vi "Authorization Write License File.vi"(8 "error in (no error)":errorcluster, 9 "Authorization":T1, 10 "Hardware ID":string, 11 "Spartan License File Path":path) -> (0 "error out":errorcluster)   [LabVIEW 2011]
uses:
  Authorization Data.ctl
panel:
  in  "Debug? (f)":bool
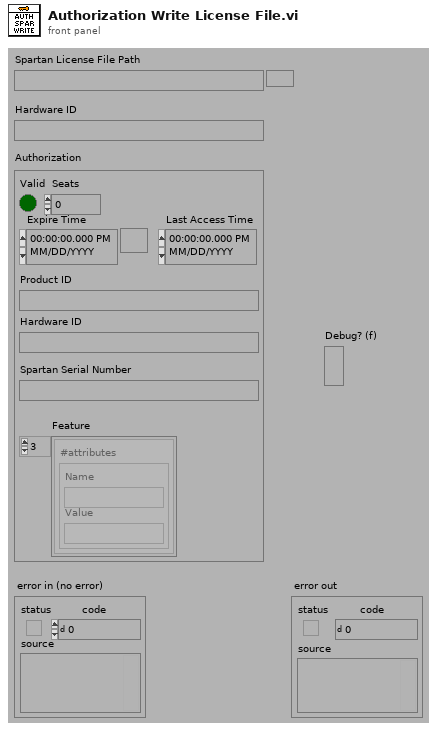
[diagram p1: front panel]
types:
  T1 = typedef "Authorization Data.ctl" = cluster{"Valid":bool, "Seats":i32, "Expire Time":timestamp, "Last Access Time":timestamp, "Product ID":string, "Hardware ID":string, "Spartan Serial Number":string, "Feature":cluster{"#attributes":cluster{"Name":string, "Value":string}}[]}
  T2 = cluster{"#attributes":cluster{"Name":string, "Value":string}}[]
  T3 = cluster{"#attributes":cluster{"Name":string, "Value":string}}
  T4 = enum16{"open", "replace", "create", "open or create", "replace or create", "replace or create with confirmation"}
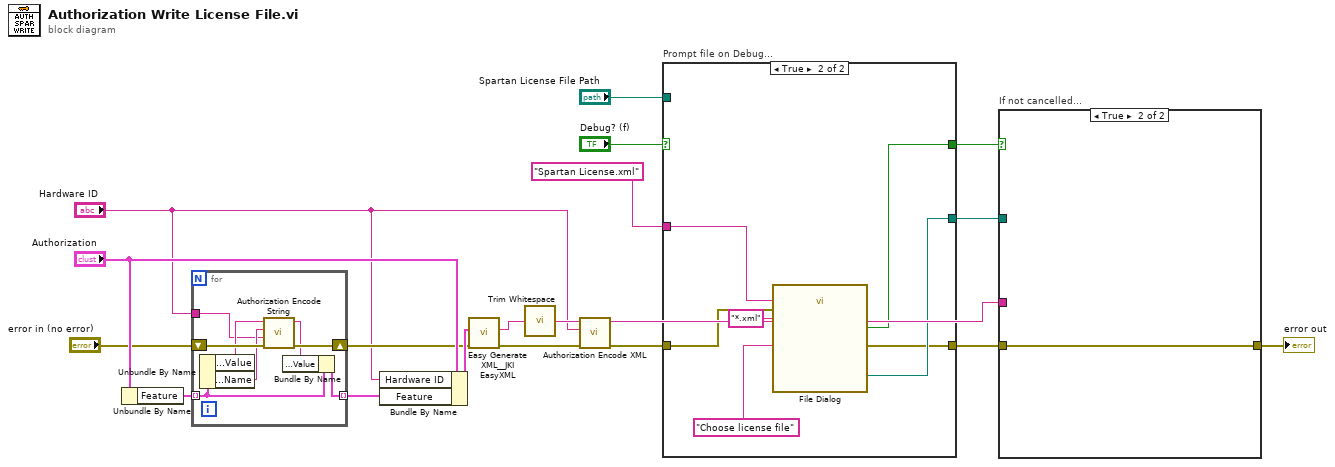
[diagram p0: block diagram]
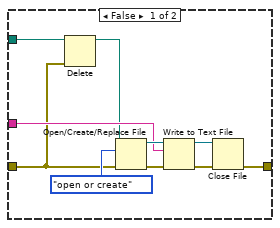
[diagram p2: hidden frame]
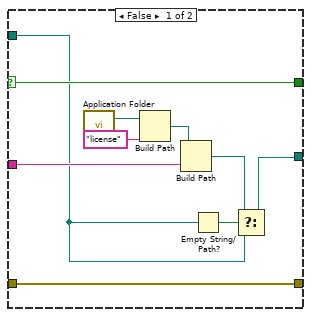
[diagram p3: hidden frame]
diagram:
  n1 = Unbundle By Name("Authorization") -> ("Feature"=w11:T2)
  n2 = for {
    tunnel: w11 -> [w26] mode=indexing
    tunnel: [w25] -> w10 mode=indexing
    shift-right: [w23] -> _
    shift-left: "error in (no error)" -> [w24]
    tunnel: "Hardware ID" -> [w19]
    n3 = Unbundle By Name(w26) -> ("#attributes.Value"=w21:string, "#attributes.Name"=w22:string)
    n4 = call "Authorization Encode String.vi"("error in (no error)"=w24, "Volume Serial Number"=w19, "Property Name"=w22, "Decoded String"=w21) -> ("error out"=w23:errorcluster, "Encoded String"=w20:string)  [unwired: 6 in]
    n5 = Bundle By Name(cluster=w26, "#attributes.Value"=w20) -> (w25:T3)
  }
  n6 = Bundle By Name(cluster="Authorization", "Hardware ID"="Hardware ID", "Feature"=w10) -> (w15:T1)
  n7 = call "Easy Generate XML__JKI EasyXML.vi"("error in (no error)"="error in (no error)", "LabVIEW Data"=w15) -> ("error out"=w18:errorcluster, "XML String"=w14:string)  [unwired: 8 in]
  n8 = call <vilib>:"Trim Whitespace.vi"("string"=w14) -> ("trimmed string"=w13:string)  [unwired: 1 in]
  n9 = call "Authorization Encode XML.vi"("error in (no error)"=w18, "Volume Serial Number"="Hardware ID", "Decoded XML String"=w13) -> ("error out"=w4:errorcluster, "Encoded XML String"=w16:string)  [unwired: 7 in]
  n10 = case "Prompt file on Debug..." shown="True" "Debug? (f)" {
    selector: "Debug? (f)" -> [w35 _]
    tunnel: [w28 w43] -> w2
    tunnel: "Spartan License.xml" ("Relative Path (\"\" - Folder)") -> [w31 w40]
    tunnel: [w36 w38] -> w3
    tunnel: w4 -> [w36 w39]
    tunnel: [w35 w37] -> w5
    tunnel: "Spartan License File Path" -> [w27 _]
    frame False {
      n11 = call "Application Folder.vi"() -> ("Application Folder"=w34:path)  [unwired: 3 in]
      n12 = Build Path(base path=w34, name or relative path="license" ("Relative Path (\"\" - Folder)")) -> (appended path=w32:path)
      n13 = Build Path(base path=w32, name or relative path=w31) -> (appended path=w29:path)
      n14 = Empty String/Path?(string/path=w27) -> (empty?=w30:bool)
      n15 = Select(t=w29, s=w30, f=w27) -> (s? t:f=w28:path)
    }
    frame True {
      n16 = call "File Dialog"("prompt"="Choose license file", "default name"=w40, "error in"=w39, "pattern (all files)"="*.xml") -> ("selected path"=w43:path, "cancelled"=w37:bool, "error out"=w38:errorcluster)  [unwired: 8 in, 1 out]
    }
  }
  n17 = case "If not cancelled..." shown="True" w5 {
    tunnel: [w51 w54] -> w17
    tunnel: w16 -> [w48 _]
    tunnel: w3 -> [w46 w54]
    tunnel: w2 -> [w44 _]
    frame False {
      n18 = Delete(path (use dialog)=w44, error in=w46) -> (deleted path=w45:path)  [unwired: 3 in, 2 out]
      n19 = Open/Create/Replace File(file path (use dialog)=w45, error in=w46, operation (0:open)=T4."open or create") -> (refnum out=w49:refnum<file>, error out=w53:errorcluster)  [unwired: 3 in, 1 out]
      n20 = Write to Text File(file (use dialog)=w49, text=w48, error in=w53) -> (refnum out=w50:refnum<file>, error out=w52:errorcluster)  [unwired: 1 in, 1 out]
      n21 = Close File(refnum=w50, error in=w52) -> (error out=w51:errorcluster)  [unwired: 1 out]
    }
    frame True {
    }
  }
  "error out" <- w17
